vi "Normalize PSD Signals.vi"(1 "Raw PSD voltages\n(Vc sum, Va sum, Va diff, Vc diff)":dbl[][](array[numeric])) -> (0 "Normalized positions\n(Vc, Va, sum)":dbl[][](array[numeric]))   [LabVIEW 2010]
panel:
  # "INPUTS:"
  # "OUTPUTS:"
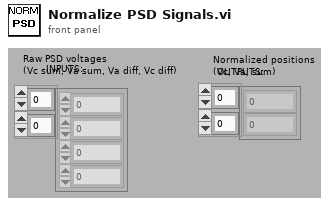
[diagram p1: front panel]
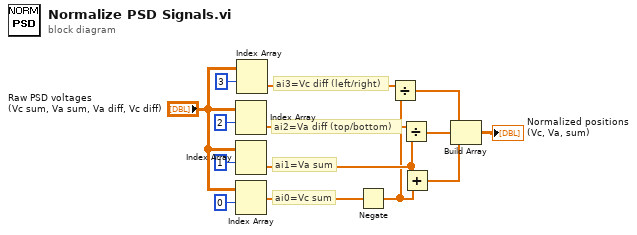
[diagram p0: block diagram]
diagram:
  # "ai3=Vc diff (left/right)"
  # "ai2=Va diff (top/bottom)"
  # "ai1=Va sum"
  # "ai0=Vc sum"
  n1 = Index Array(array="Raw PSD voltages\n(Vc sum, Va sum, Va diff, Vc diff)", index (row)=2 ("index")) -> (element=w11:dbl[])  [unwired: 1 in]
  n2 = Index Array(array="Raw PSD voltages\n(Vc sum, Va sum, Va diff, Vc diff)", index (row)=1 ("index")) -> (element=w3:dbl[])  [unwired: 1 in]
  n3 = Index Array(array="Raw PSD voltages\n(Vc sum, Va sum, Va diff, Vc diff)", index (row)=0 ("index")) -> (element=w10:dbl[])  [unwired: 1 in]
  n4 = Index Array(array="Raw PSD voltages\n(Vc sum, Va sum, Va diff, Vc diff)", index (row)=3 ("index")) -> (element=w9:dbl[])  [unwired: 1 in]
  n5 = Negate(x=w10) -> (-x=w2:dbl[])
  n6 = Divide(x=w9, y=w2) -> (x/y=w12:dbl[])
  n7 = Divide(x=w11, y=w3) -> (x/y=w13:dbl[])
  n8 = Add(x=w3, y=w2) -> (x+y=w1:dbl[])
  n9 = Build Array(w12, w13, w1) -> (→"Normalized positions\n(Vc, Va, sum)":dbl[][])
